vi "Wire Return Param.vi"(10 "Proto VI Ref":refnum<vi>, 11 "Abstract Param Writer in":refnum<class "Abstract Param Writer.lvclass">) -> (3 "Abstract Param Writer out":refnum<class "Abstract Param Writer.lvclass">)   [LabVIEW 2013, in "Abstract Param Writer.lvclass"]
doc: "Copyright (c) 2016 Sze Howe Koh\n\nThis Source Code Form is subject to the terms of the Mozilla Public License, v. 2.0. If a copy of the MPL was not distributed with this file, You can obtain one at http://mozilla.org/MPL/2.0/."
uses:
  Abstract Param Writer.lvclass
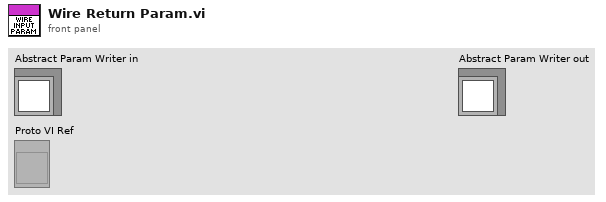
[diagram p1: front panel]
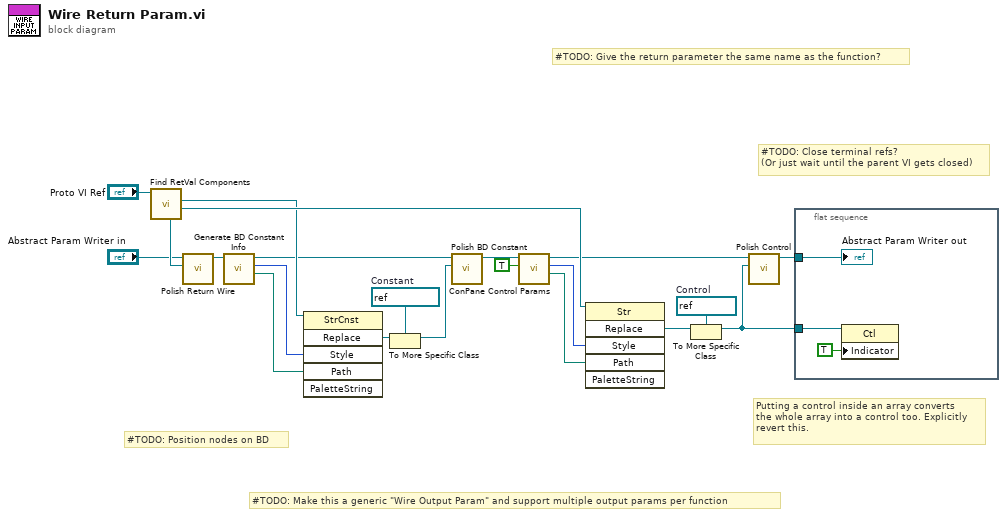
[diagram p0: block diagram]
diagram:
  w12 = refnum<vi> refnum  # Constant
  w18 = refnum<vi> refnum  # Control
  # "#TODO: Give the return parameter the same name as the function?"
  # "Putting a control inside an array converts\nthe whole array into a control too. Explicitly\nrevert this."
  # "#TODO: Make this a generic \"Wire Output Param\" and support multiple output params per function"
  # "#TODO: Close terminal refs?\n(Or just wait until the parent VI gets closed)"
  # "#TODO: Position nodes on BD"
  n1 = call "Find RetVal Components.vi"("Proto Method VI"="Proto VI Ref") -> ("Indicator"=w16:refnum<vi>, "Data Buffer"=w15:refnum<vi>, "Wire"=w9:refnum<vi>)  [unwired: 6 in, 2 out]
  n2 = call-dynamic "Polish Return Wire.vi"("Return Wire"=w9, "Abstract Param Writer in"="Abstract Param Writer in") -> ("Abstract Param Writer out"=w2:refnum<class "Abstract Param Writer.lvclass">)  [unwired: 9 in]
  n3 = call-dynamic "Generate BD Constant Info.vi"("Abstract Param Writer in"=w2) -> ("Path"=w13:path, "Style"=w14:i32, "Abstract Param Writer out"=w8:refnum<class "Abstract Param Writer.lvclass">)  [unwired: 8 in]
  n4 = invoke class="StrCnst" method="Replace"(reference=w15, "Style"=w14, "Path"=w13) -> ("Replace"=w11:refnum<vi>)  [unwired: 3 in, 5 out]
  n5 = To More Specific Class(target class=w12, reference=w11) -> (specific class reference=w10:refnum<vi>)  [unwired: 1 in, 1 out]
  n6 = call-dynamic "Polish BD Constant.vi"("BD Const"=w10, "Abstract Param Writer in"=w8) -> ("Abstract Param Writer out"=w4:refnum<class "Abstract Param Writer.lvclass">)  [unwired: 9 in]
  n7 = call-dynamic "ConPane Control Params.vi"("Indicator? (F)"=TRUE, "Abstract Param Writer in"=w4) -> ("Path"=w20:path, "Style"=w21:i32, "Abstract Param Writer out"=w7:refnum<class "Abstract Param Writer.lvclass">)  [unwired: 7 in]
  n8 = invoke class="Str" method="Replace"(reference=w16, "Style"=w21, "Path"=w20) -> ("Replace"=w19:refnum<vi>)  [unwired: 3 in, 5 out]
  n9 = To More Specific Class(target class=w18, reference=w19) -> (specific class reference=w6:refnum<vi>)  [unwired: 1 in, 1 out]
  n10 = call-dynamic "Polish Control.vi"("Control Ref"=w6, "Abstract Param Writer in"=w7) -> ("Abstract Param Writer out"=w5:refnum<class "Abstract Param Writer.lvclass">)  [unwired: 9 in]
  n11 = flat-sequence {
    tunnel: w6 -> [w23]
    tunnel: w5 -> [w22]
    frame #0 {
      n12 = property class="Ctl"(reference=w23, "Indicator"=TRUE) -> ()  [unwired: 1 in, 2 out]
      "Abstract Param Writer out" <- w22
    }
  }
